vi "calc.vi"() -> ()   [LabVIEW 2011]
uses:
  global_vars.vi
  <vilib>/Utility/file.llb/Write To Spreadsheet File (DBL).vi
panel:
  out "i32_ar_displacement":dbl[][](array[numeric])
  in  "b_calc_all":bool
  out "calculating":bool
  in  "calc \ndisplacement":bool
  in  "file path (dialog if empty)":path
  in  "dbl_gamma_correction":dbl=1.0
  in  "dbl_noise_threshold":dbl=5000.0
  in  "update global variables":bool
  in  "safety margin":i32=5
  out "u8_ar_noise_mask":u8[][](array[numeric])
  in  "Tab Control":T1(tab)
  out "img_dist_input":T2(plugin-control)
  out "img_orig_input":T2(plugin-control)
  in  "i32_sel_input_image":i32
  in  "select row input":i32(slide) scale=-1.1..1023.0
  out "input_line_plot":dbl[][](graph)
  out "noise_mask_line_plot":u8[](graph)
  in  "select row noise map":i32(slide) scale=-1.1..1023.0
  out "last px":i32
  out "first px":i32
  out "img_noise_mask":T2(plugin-control)
  out "i32_First/last px":i32[][](graph)
  out "lineplot phasemap":dbl[][](graph)
  in  "select row phasemap":i32(slide) scale=-1.1..1023.0
  out "img_dist_phaseMap":T2(plugin-control)
  out "img_orig_masked_with_dist":T2(plugin-control)
  out "img_dist_unwrap":T2(plugin-control)
  out "img_orig_unwrap":T2(plugin-control)
  in  "select row unwrapped":i32(slide) scale=-1.1..1023.0
  out "lineplot unwrapped":dbl[][](graph)
  out "graph_displacement":dbl[][](graph)
  in  "select row displacement":i32(slide) scale=-1.1..1023.0
  out "lineplot displacement 2":dbl[](graph)
  in  "save data":bool
  in  "calc \nunwrapped\nphase map":bool
  out "Y Resolution":i32
  out "X Resolution":i32
  in  "update_cor":bool
  out "path_dist_files":path[](array[path])=[path "X:/Cloud Drives/Dropbox/Europhotonics/FringeMan/Image Storage/02_07/x-direction/dist/12_56_10-5.00fringes_0of4__capt_.png", path "X:/Cloud Drives/Dropbox/Europhotonics/FringeMan/Image Storage/02_07/x-direction/dist/12_56_10-5.00fringes_1of4__capt_.png", path "X:/Cloud Drives/Dropbox/Europhotonics/FringeMan/Image Storage/02_07/x-direction/dist/12_56_10-5.00fringes_2of4__capt_.png", path "X:/Cloud Drives/Dropbox/Europhotonics/FringeMan/Image Storage/02_07/x-direction/dist/12_56_10-5.00fringes_3of4__capt_.png"]
  out "path_orig_files":path[](array[path])=[path "X:/Cloud Drives/Dropbox/Europhotonics/FringeMan/Image Storage/02_07/x-direction/orig/12_56_10-5.00fringes_0of4__original_.png", path "X:/Cloud Drives/Dropbox/Europhotonics/FringeMan/Image Storage/02_07/x-direction/orig/12_56_10-5.00fringes_1of4__original_.png", path "X:/Cloud Drives/Dropbox/Europhotonics/FringeMan/Image Storage/02_07/x-direction/orig/12_56_10-5.00fringes_2of4__original_.png", path "X:/Cloud Drives/Dropbox/Europhotonics/FringeMan/Image Storage/02_07/x-direction/orig/12_56_10-5.00fringes_3of4__original_.png"]
  in  "dbl_ar_crop_correction":dbl[](array[numeric])=[0.0, 0.0, 0.0, 0.0] caption="crop_correction"
  in  "u8_y_center_cor":i16
  in  "u8_x_center_cor":i16=-20
  in  "radius correction":i16=-30
  out "u8_ar_orig_phasemap":dbl[][](array[numeric])
  out "dbl_pxar_orig_unwrap":dbl[][](array[numeric])
  out "dbl_pxar_dist_unwrap":dbl[][](array[numeric])
  out "u8_pxar_orig":u8[][][](array[numeric])
  in  "read orig":bool
  in  "read dist":bool
  out "u8_ar_dist_phasemap":dbl[][](array[numeric])
  in  "calculate \nphase map":bool
  out "u8_pxar_dist":u8[][][](array[numeric])
  in  "Stop Button":bool
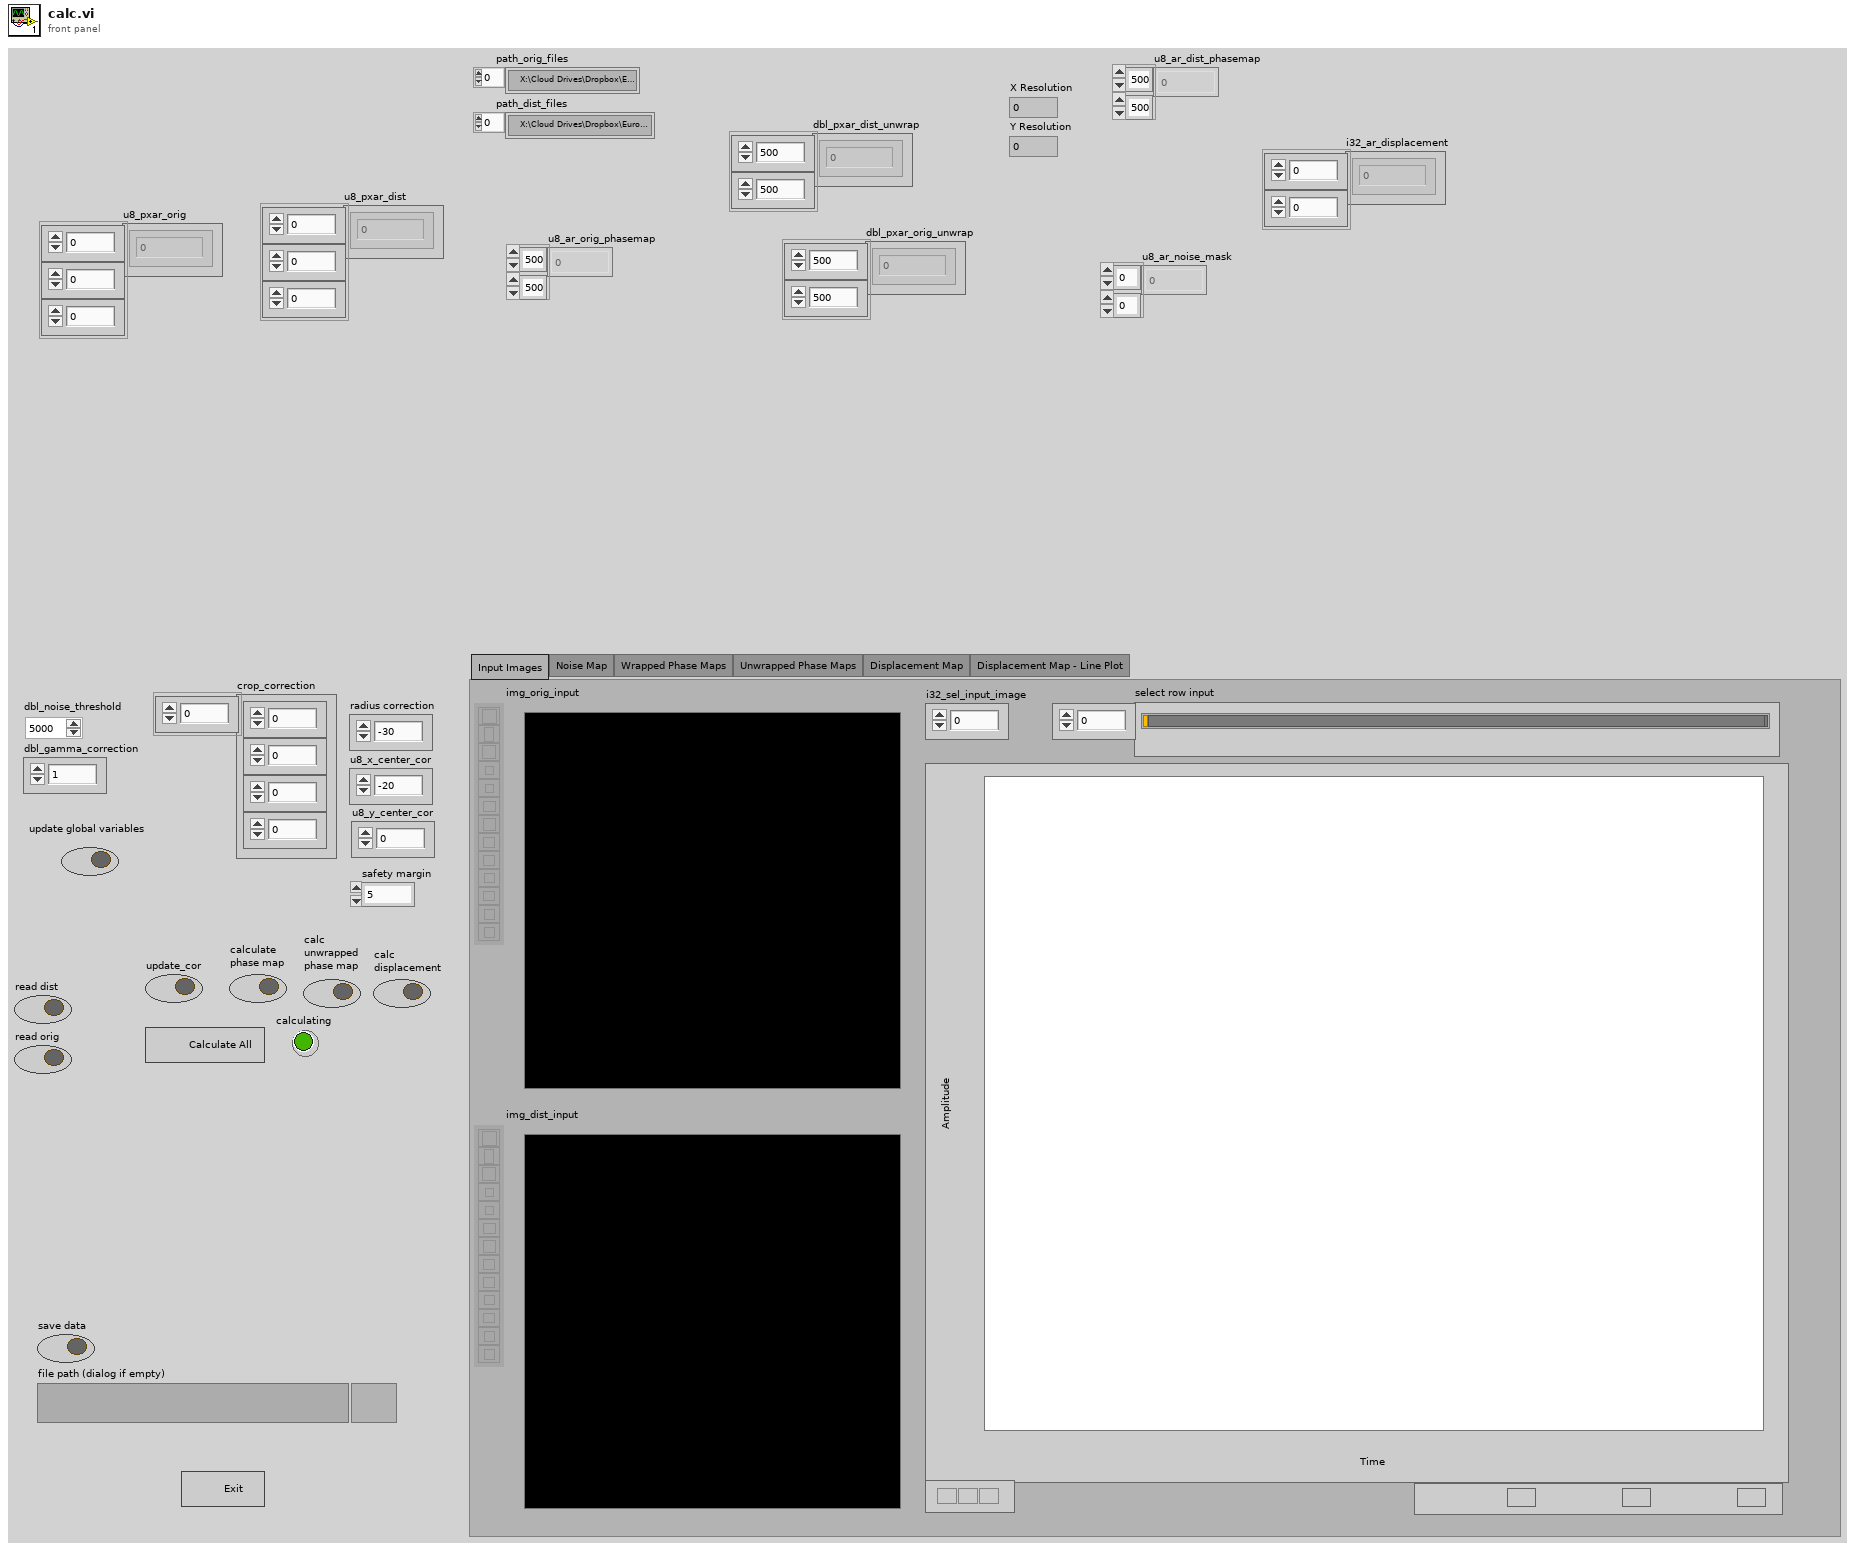
[diagram p1: front panel]
types:
  T1 = enum32{"Input Images", "Noise Map", "Wrapped Phase Maps", "Unwrapped Phase Maps", "Displacement Map", "Displacement Map - Line Plot"}
  T2 = typedef "IMAQ Image.ctl" = refnum<image>
  T3 = cluster{"radius correction":i16, "u8_x_center_cor":i16, "u8_y_center_cor":i16}
  T4 = typedef "Image Type" = u32
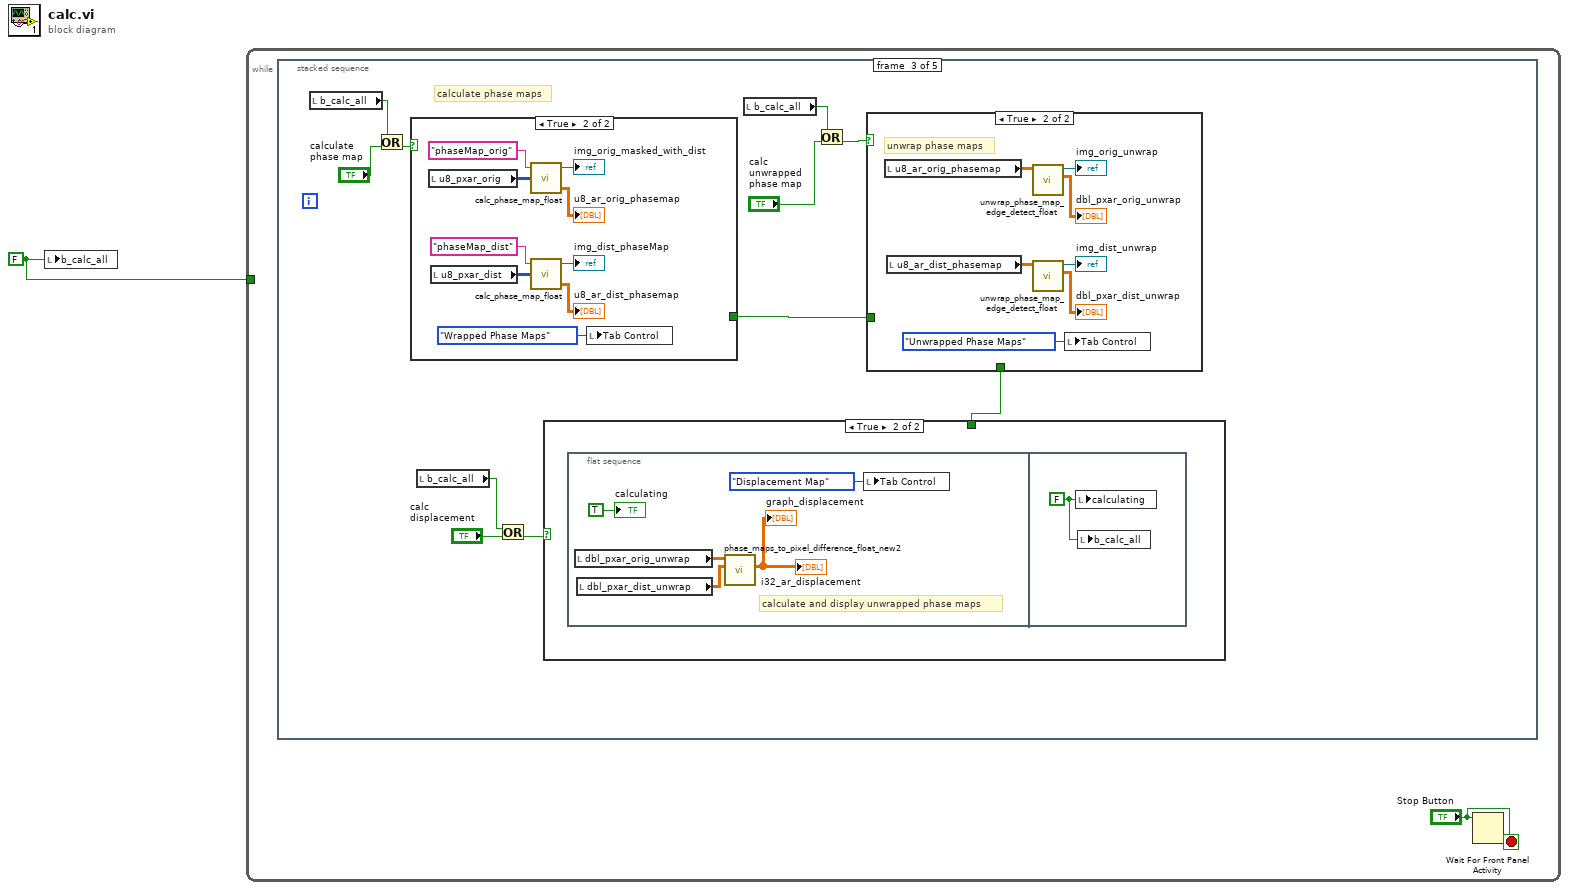
[diagram p0: block diagram]
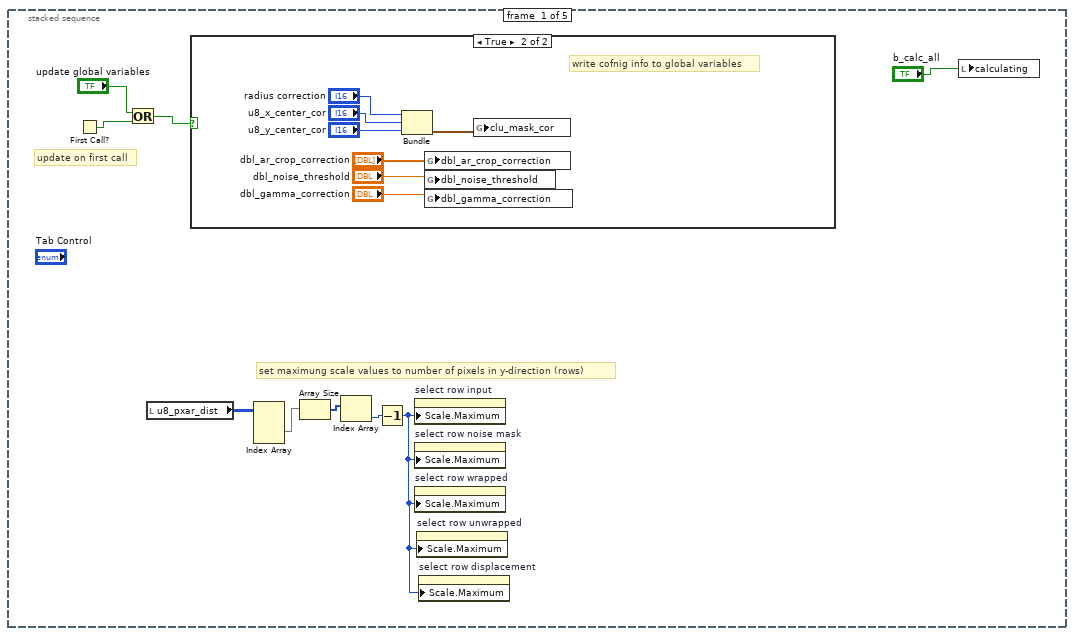
[diagram p2: hidden frame]
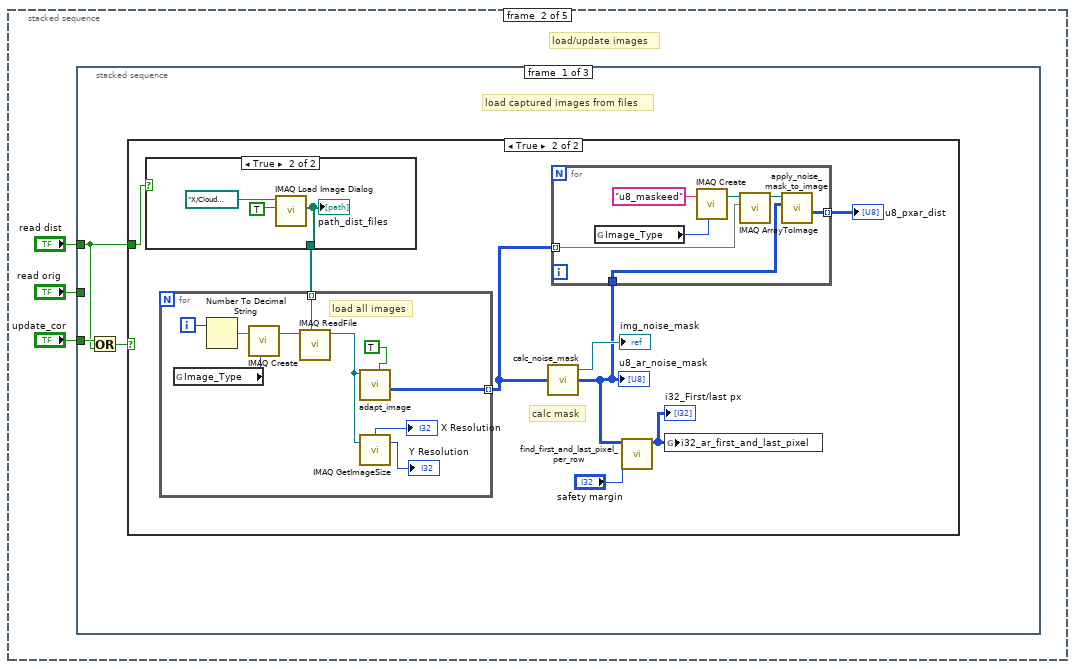
[diagram p4: hidden frame]
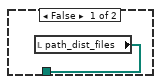
[diagram p6: hidden frame]
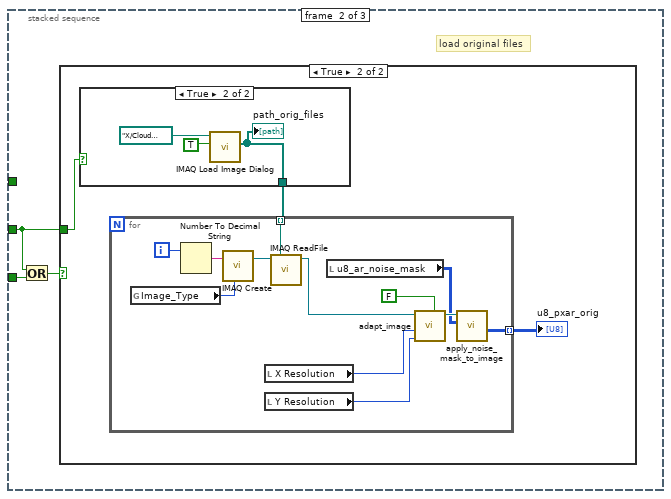
[diagram p7: hidden frame]
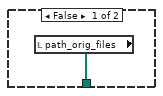
[diagram p9: hidden frame]
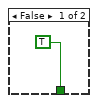
[diagram p12: hidden frame]
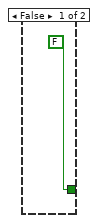
[diagram p13: hidden frame]
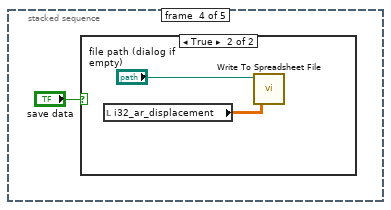
[diagram p14: hidden frame]
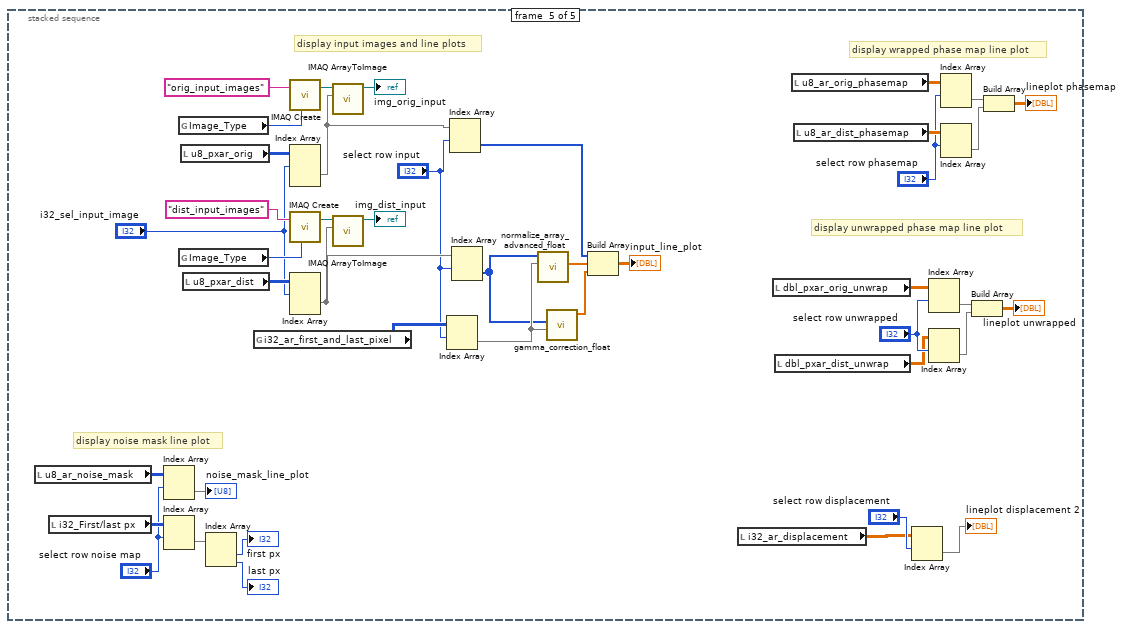
[diagram p16: hidden frame]
diagram:
  w1 = FALSE ("b_calculate all")
  n1 = local write "b_calc_all"(w1) -> ()
  n2 = while {
    tunnel: w1 -> [_]
    stop <- "Stop Button" stop-if-true
    n3 = stacked-sequence {
      frame #0 {
        # "set maximung scale values to number of pixels in y-direction (rows)"
        # "update on first call"
        n4 = First Call?() -> (First Call?: T/F=w9:bool)
        n5 = Or(x="update global variables", y=w9) -> (x .or. y?=w10:bool)
        n6 = local read "u8_pxar_dist"() -> (w7:u8[][][])
        n7 = case shown="True" w10 {
          frame False {
          }
          frame True {
            # "write cofnig info to global variables"
            n8 = Bundle("radius correction"="radius correction", "u8_x_center_cor"="u8_x_center_cor", "u8_y_center_cor"="u8_y_center_cor") -> (w18:T3)  [unwired: 1 in]
            n9 = global write "global_vars.vi" "dbl_ar_crop_correction"("dbl_ar_crop_correction") -> ()
            n10 = global write "global_vars.vi" "dbl_noise_threshold"("dbl_noise_threshold") -> ()
            n11 = global write "global_vars.vi" "dbl_gamma_correction"("dbl_gamma_correction") -> ()
            n12 = global write "global_vars.vi" "clu_mask_cor"(w18) -> ()
          }
        }
        n13 = Index Array(array=w7) -> (element=w8:u8[][])  [unwired: 3 in]
        n14 = Array Size(array=w8) -> (size(s)=w6:i32[])
        n15 = Index Array(array=w6) -> (element=w5:i32)  [unwired: 1 in]
        n16 = Decrement(x=w5) -> (x-1=w4:i32)
        n17 = property on="select row input" class="Slide (strict)"("Scale.Maximum"=w4) -> ()  [unwired: 2 in, 2 out]
        n18 = property on="select row noise mask" class="Slide (strict)"("Scale.Maximum"=w4) -> ()  [unwired: 2 in, 2 out]
        n19 = property on="select row wrapped" class="Slide (strict)"("Scale.Maximum"=w4) -> ()  [unwired: 2 in, 2 out]
        n20 = property on="select row unwrapped" class="Slide (strict)"("Scale.Maximum"=w4) -> ()  [unwired: 2 in, 2 out]
        n21 = property on="select row displacement" class="Slide (strict)"("Scale.Maximum"=w4) -> ()  [unwired: 2 in, 2 out]
        n22 = local write "calculating"("b_calc_all") -> ()
      }
      frame #1 {
        # "load/update images"
        n23 = stacked-sequence {
          tunnel: "update_cor" -> [w24 w55 _]
          tunnel: "read dist" -> [w22 _ _]
          tunnel: "read orig" -> [_ w54 _]
          frame #0 {
            # "load captured images from files"
            n24 = Or(x=w24, y=w22) -> (x .or. y?=w23:bool)
            n25 = case shown="True" w23 {
              tunnel: w22 -> [_ w31]
              frame False {
              }
              frame True {
                # "calc mask"
                n26 = case shown="True" w31 {
                  tunnel: [w40 w43] -> w32
                  frame False {
                    n27 = local read "path_dist_files"() -> (w40:path[])
                  }
                  frame True {
                    n28 = call "IMAQ Load Image Dialog"("Multiple Files? (No)"=TRUE, "Start Path"=path "X:/Cloud Drives/Dropbox/Europhotonics/FringeMan/Image Storage") -> ("Paths"=w43:path[])  [unwired: 7 in, 2 out]
                    "path_dist_files" <- w43
                  }
                }
                n29 = for {
                  tunnel: w32 -> [w49] mode=indexing
                  tunnel: [w45] -> w26 mode=indexing
                  i -> [w53]
                  # "load all images"
                  n30 = global read "global_vars.vi" "Image_Type"() -> (w50:T4)
                  n31 = Number To Decimal String(number=w53) -> (decimal integer string=w52:string)  [unwired: 1 in]
                  n32 = call "IMAQ Create"("Image Name"=w52, "Image Type"=w50) -> ("New Image"=w51:T2)  [unwired: 2 in, 2 out]
                  n33 = call "IMAQ ReadFile"("File Path"=w49, "Image"=w51) -> ("Image Out"=w46:T2)  [unwired: 5 in, 4 out]
                  n34 = call "adapt_image.vi"("captured image?"=TRUE, "orig_imageIn"=w46) -> ("adapted image px array"=w45:u8[][])  [unwired: 8 in, 1 out]
                  n35 = call "IMAQ GetImageSize"("Image"=w46) -> ("Y Resolution"=→"Y Resolution":i32, "X Resolution"=→"X Resolution":i32)  [unwired: 3 in, 1 out]
                }
                n36 = call "calc_noise_mask.vi"("u8_ar_image_pixel_array"=w26) -> ("u8_ar_noise_mask"=w25:u8[][], "img_noise mask"=→"img_noise_mask":T2)  [unwired: 3 in]
                "u8_ar_noise_mask" <- w25
                n37 = for {
                  tunnel: w26 -> [w39] mode=indexing
                  tunnel: [w34] -> w27 mode=indexing
                  tunnel: w25 -> [w33]
                  n38 = global read "global_vars.vi" "Image_Type"() -> (w38:T4)
                  n39 = call "IMAQ Create"("Image Name"="u8_maskeed", "Image Type"=w38) -> ("New Image"=w36:T2)  [unwired: 2 in, 2 out]
                  n40 = call "IMAQ ArrayToImage"("Image Pixels (U8)"=w39, "Image"=w36) -> ("Image Out"=w35:T2)  [unwired: 8 in, 1 out]
                  n41 = call "apply_noise_mask_to_image.vi"("u8_ar_noise_mask in"=w33, "Refnum in"=w35) -> ("Image Pixels (U8)"=w34:u8[][])  [unwired: 7 in, 2 out]
                }
                "u8_pxar_dist" <- w27
                n42 = call "find_first_and_last_pixel_per_row.vi"("safety margin"="safety margin", "u8_ar_mask"=w25) -> ("i32_ar_first_and_last_pixel"=w28:i32[][])  [unwired: 9 in]
                "i32_First/last px" <- w28
                n43 = global write "global_vars.vi" "i32_ar_first_and_last_pixel"(w28) -> ()
              }
            }
          }
          frame #1 {
            # "load original files"
            n44 = Or(x=w54, y=w55) -> (x .or. y?=w56:bool)
            n45 = case shown="True" w56 {
              tunnel: w54 -> [_ w58]
              frame False {
              }
              frame True {
                n46 = case shown="True" w58 {
                  tunnel: [w60 w62] -> w59
                  frame False {
                    n47 = local read "path_orig_files"() -> (w60:path[])
                  }
                  frame True {
                    n48 = call "IMAQ Load Image Dialog"("Multiple Files? (No)"=TRUE, "Start Path"=path "X:/Cloud Drives/Dropbox/Europhotonics/FringeMan/Image Storage") -> ("Paths"=w62:path[])  [unwired: 7 in, 2 out]
                    "path_orig_files" <- w62
                  }
                }
                n49 = for {
                  tunnel: w59 -> [w75] mode=indexing
                  tunnel: [w65] -> w57 mode=indexing
                  i -> [w71]
                  n50 = global read "global_vars.vi" "Image_Type"() -> (w72:T4)
                  n51 = Number To Decimal String(number=w71) -> (decimal integer string=w74:string)  [unwired: 1 in]
                  n52 = call "IMAQ Create"("Image Name"=w74, "Image Type"=w72) -> ("New Image"=w73:T2)  [unwired: 2 in, 2 out]
                  n53 = local read "X Resolution"() -> (w69:i32)
                  n54 = local read "Y Resolution"() -> (w68:i32)
                  n55 = call "IMAQ ReadFile"("File Path"=w75, "Image"=w73) -> ("Image Out"=w70:T2)  [unwired: 5 in, 4 out]
                  n56 = local read "u8_ar_noise_mask"() -> (w64:u8[][])
                  n57 = call "adapt_image.vi"("captured image?"=FALSE, "captImage_Y_Resolution"=w68, "captImage_X_Resolution"=w69, "orig_imageIn"=w70) -> ("adapted image"=w66:T2)  [unwired: 6 in, 1 out]
                  n58 = call "apply_noise_mask_to_image.vi"("u8_ar_noise_mask in"=w64, "Refnum in"=w66) -> ("Image Pixels (U8)"=w65:u8[][])  [unwired: 7 in, 2 out]
                }
                "u8_pxar_orig" <- w57
              }
            }
          }
          frame #2 {
          }
        }
      }
      frame #2 {
        # "calculate phase maps"
        n59 = local read "b_calc_all"() -> (w78:bool)
        n60 = Or(x=w78, y="calculate \nphase map") -> (x .or. y?=w81:bool)
        n61 = case shown="True" w81 {
          tunnel: [FALSE _] -> w84
          frame False {
          }
          frame True {
            n62 = local read "u8_pxar_orig"() -> (w105:u8[][][])
            n63 = local read "u8_pxar_dist"() -> (w109:u8[][][])
            n64 = call "calc_phase_map_float.vi"("u8_ar_image_pixel_array"=w105, "image name"="phaseMap_orig" ("String")) -> ("raw phase map array"=→"u8_ar_orig_phasemap":dbl[][], "phase map"=→"img_orig_masked_with_dist":T2)  [unwired: 2 in]
            n65 = call "calc_phase_map_float.vi"("u8_ar_image_pixel_array"=w109, "image name"="phaseMap_dist" ("String")) -> ("raw phase map array"=→"u8_ar_dist_phasemap":dbl[][], "phase map"=→"img_dist_phaseMap":T2)  [unwired: 2 in]
            n66 = local write "Tab Control"(T1."Wrapped Phase Maps" ("Tab Control")) -> ()
          }
        }
        n67 = local read "b_calc_all"() -> (w76:bool)
        n68 = Or(x=w76, y="calc \ndisplacement") -> (x .or. y?=w79:bool)
        n69 = local read "b_calc_all"() -> (w77:bool)
        n70 = Or(x=w77, y="calc \nunwrapped\nphase map") -> (x .or. y?=w80:bool)
        n71 = case shown="True" w80 {
          tunnel: w84 -> [_ _]
          tunnel: [TRUE _] -> w82
          frame False {
          }
          frame True {
            # "unwrap phase maps"
            n72 = local read "u8_ar_orig_phasemap"() -> (w97:dbl[][])
            n73 = local read "u8_ar_dist_phasemap"() -> (w98:dbl[][])
            n74 = call "unwrap_phase_map_edge_detect_float.vi"("u8_ar_dist_phasemap"=w97) -> ("df_ar_unwrapped_px_ar"=→"dbl_pxar_orig_unwrap":dbl[][], "Refnum out"=→"img_orig_unwrap":T2)  [unwired: 9 in]
            n75 = call "unwrap_phase_map_edge_detect_float.vi"("u8_ar_dist_phasemap"=w98) -> ("df_ar_unwrapped_px_ar"=→"dbl_pxar_dist_unwrap":dbl[][], "Refnum out"=→"img_dist_unwrap":T2)  [unwired: 9 in]
            n76 = local write "Tab Control"(T1."Unwrapped Phase Maps" ("Tab Control")) -> ()
          }
        }
        n77 = case shown="True" w79 {
          tunnel: w82 -> [_ _]
          frame False {
          }
          frame True {
            n78 = flat-sequence {
              frame #0 {
                # "calculate and display unwrapped phase maps"
                n79 = local read "dbl_pxar_orig_unwrap"() -> (w89:dbl[][])
                n80 = local read "dbl_pxar_dist_unwrap"() -> (w90:dbl[][])
                n81 = call "phase_maps_to_pixel_difference_float_new2.vi"("dist phase map"=w90, "oirg phase map"=w89) -> ("displacement map 2"=→"graph_displacement" →"i32_ar_displacement":dbl[][])  [unwired: 8 in, 1 out]
                n82 = local write "Tab Control"(T1."Displacement Map" ("Tab Control")) -> ()
                "calculating" <- TRUE
              }
              frame #1 {
                w92 = FALSE
                n83 = local write "calculating"(w92) -> ()
                n84 = local write "b_calc_all"(w92) -> ()
              }
            }
          }
        }
      }
      frame #3 {
        n85 = case shown="True" "save data" {
          frame False {
          }
          frame True {
            n86 = local read "i32_ar_displacement"() -> (w113:dbl[][])
            n87 = call-poly <vilib>:"Write To Spreadsheet File.vi"("2D data"=w113, "file path (dialog if empty)"="file path (dialog if empty)") -> ()  [unwired: 6 in, 1 out]
          }
        }
      }
      frame #4 {
        # "display unwrapped phase map line plot"
        # "display noise mask line plot"
        # "display wrapped phase map line plot"
        # "display input images and line plots"
        n88 = local read "u8_ar_noise_mask"() -> (w150:u8[][])
        n89 = local read "i32_First/last px"() -> (w145:i32[][])
        n90 = Index Array(array=w150, index (row)="select row noise map") -> (element=→"noise_mask_line_plot":u8[])  [unwired: 1 in]
        n91 = Index Array(array=w145, index (row)="select row noise map") -> (element=w146:i32[])  [unwired: 1 in]
        n92 = global read "global_vars.vi" "Image_Type"() -> (w140:T4)
        n93 = global read "global_vars.vi" "Image_Type"() -> (w137:T4)
        n94 = local read "u8_pxar_orig"() -> (w141:u8[][][])
        n95 = local read "u8_pxar_dist"() -> (w142:u8[][][])
        n96 = Index Array(array=w146) -> (element #1=→"first px":i32, element #2=→"last px":i32)  [unwired: 2 in]
        n97 = global read "global_vars.vi" "i32_ar_first_and_last_pixel"() -> (w131:i32[][])
        n98 = call "IMAQ Create"("Image Name"="orig_input_images", "Image Type"=w140) -> ("New Image"=w135:T2)  [unwired: 2 in, 2 out]
        n99 = Index Array(array=w141, index (dim 0)="i32_sel_input_image") -> (element=w132:u8[][])  [unwired: 2 in]
        n100 = call "IMAQ Create"("Image Name"="dist_input_images", "Image Type"=w137) -> ("New Image"=w136:T2)  [unwired: 2 in, 2 out]
        n101 = Index Array(array=w142, index (dim 0)="i32_sel_input_image") -> (element=w143:u8[][])  [unwired: 2 in]
        n102 = call "IMAQ ArrayToImage"("Image Pixels (U8)"=w132, "Image"=w135) -> ("Image Out"=→"img_orig_input":T2)  [unwired: 8 in, 1 out]
        n103 = call "IMAQ ArrayToImage"("Image Pixels (U8)"=w143, "Image"=w136) -> ("Image Out"=→"img_dist_input":T2)  [unwired: 8 in, 1 out]
        n104 = Index Array(array=w131, index (row)="select row input") -> (element=w127:i32[])  [unwired: 1 in]
        n105 = Index Array(array=w132, index (row)="select row input") -> (element=w125:u8[])  [unwired: 1 in]
        n106 = Index Array(array=w143, index (row)="select row input") -> (element=w123:u8[])  [unwired: 1 in]
        n107 = call "normalize_array_advanced_float.vi"("i32_ar_first_and_last_pixel"=w127, "unwrapped array"=w123) -> ("i16_normalized unwrapped array"=w124:dbl[])  [unwired: 5 in, 4 out]
        n108 = call "gamma_correction_float.vi"("i32_ar_first_and_last_pixel"=w127, "u8_pxar_dist"=w123) -> ("i16_normalized unwrapped array"=w126:dbl[])  [unwired: 9 in]
        n109 = Build Array(w125, w124, w126) -> (→"input_line_plot":dbl[][])
        n110 = local read "i32_ar_displacement"() -> (w115:dbl[][])
        n111 = local read "dbl_pxar_orig_unwrap"() -> (w118:dbl[][])
        n112 = local read "dbl_pxar_dist_unwrap"() -> (w117:dbl[][])
        n113 = local read "u8_ar_orig_phasemap"() -> (w156:dbl[][])
        n114 = local read "u8_ar_dist_phasemap"() -> (w155:dbl[][])
        n115 = Index Array(array=w115, index (row)="select row displacement") -> (element=→"lineplot displacement 2":dbl[])  [unwired: 1 in]
        n116 = Index Array(array=w118, index (row)="select row unwrapped") -> (element=w122:dbl[])  [unwired: 1 in]
        n117 = Index Array(array=w117, index (row)="select row unwrapped") -> (element=w121:dbl[])  [unwired: 1 in]
        n118 = Index Array(array=w156, index (row)="select row phasemap") -> (element=w153:dbl[])  [unwired: 1 in]
        n119 = Index Array(array=w155, index (row)="select row phasemap") -> (element=w152:dbl[])  [unwired: 1 in]
        n120 = Build Array(w122, w121) -> (→"lineplot unwrapped":dbl[][])
        n121 = Build Array(w153, w152) -> (→"lineplot phasemap":dbl[][])
      }
    }
    n122 = Wait For Front Panel Activity(3:"Stop Button") -> ()  [unwired: 2 in, 1 out]
  }
